vi "Tektronix_basic.vi"(7 "write buffer":string, 8 "error in (no error)":errorcluster, 9 "Query?":bool, 10 "Error query?":bool, 11 "VISA resource name":refnum<visa-resource-name>) -> (0 "error out":errorcluster, 1 "read buffer":string, 3 "VISA resource name out":refnum<visa-resource-name>)   [LabVIEW 2017]
uses:
  instr.lib/Tektronix TDS 200 1000 2000 Series/Tektronix TDS 200 1000 2000 Series.lvlib
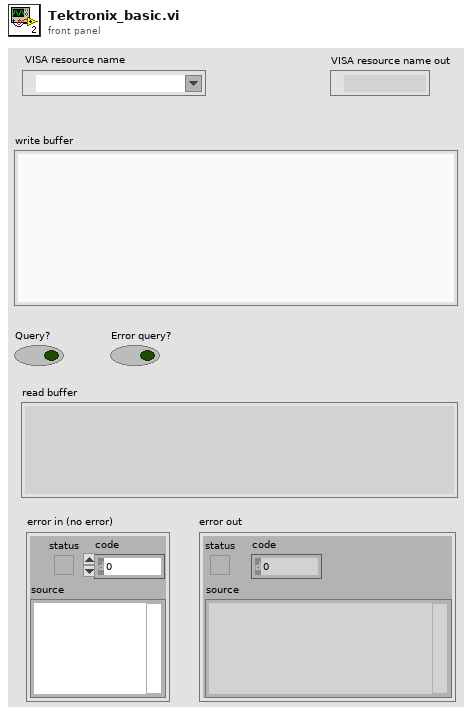
[diagram p1: front panel]
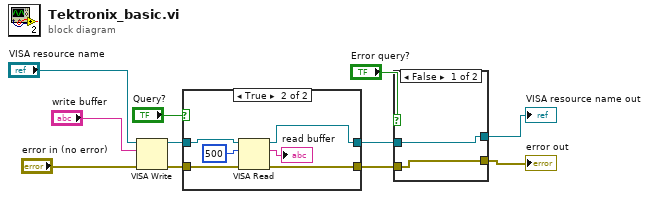
[diagram p0: block diagram]
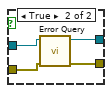
[diagram p2: hidden frame]
diagram:
  n1 = VISA Write(VISA resource name="VISA resource name", write buffer="write buffer", error in (no error)="error in (no error)") -> (VISA resource name out=w7:refnum<visa-resource-name>, error out=w8:errorcluster)  [unwired: 1 out]
  n2 = case shown="True" "Query?" {
    tunnel: w8 -> [w12 w17]
    tunnel: w7 -> [w13 w16]
    tunnel: [w12 w15] -> w3
    tunnel: [w13 w14] -> w2
    frame False {
    }
    frame True {
      n3 = VISA Read(VISA resource name=w16, byte count=u32 500, error in (no error)=w17) -> (VISA resource name out=w14:refnum<visa-resource-name>, read buffer=→"read buffer":string, error out=w15:errorcluster)  [unwired: 1 out]
    }
  }
  n4 = case shown="False" "Error query?" {
    tunnel: [w20 w25] -> w5
    tunnel: [w21 w24] -> w4
    tunnel: w3 -> [w20 w23]
    tunnel: w2 -> [w21 w22]
    frame False {
    }
    frame True {
      n5 = call "Error Query.vi"("error in (no error)"=w23, "VISA resource name"=w22) -> ("error out"=w25:errorcluster, "VISA resource name out"=w24:refnum<visa-resource-name>)  [unwired: 8 out]
    }
  }
  "error out" <- w5
  "VISA resource name out" <- w4
